vi "roboRIO v1.0 Reserve Relay.vi"(7 "Allow multiple opens?":bool, 8 "error in (no error)":errorcluster, 10 "Relay Channel List":T1) -> (0 "error out":errorcluster)   [LabVIEW 2021]
uses:
  <vilib>/myRIO/Common/Instrument Driver Framework/roboRIO v1.0/Relay/typedefs/Relay Channels List.ctl
  <vilib>/myRIO/Common/Instrument Driver Framework/roboRIO v1.0/Relay/typedefs/Relay Channels Enum.ctl
  <vilib>/myRIO/Common/Instrument Driver Framework/roboRIO v1.0/Resource Manager/vis/roboRIO v1.0 Reserve Channel.vi
  <vilib>/myRIO/Common/Instrument Driver Framework/roboRIO v1.0/Resource Manager/vis/roboRIO v1.0 Unreserve Channel.vi
  <vilib>/myRIO/Common/Instrument Driver Framework/roboRIO v1.0/Resource Manager/vis/roboRIO v1.0 Build Mutex Name.vi
  <vilib>/myRIO/Common/Instrument Driver Framework/Utilities/vis/IO Manager.vi
  <vilib>/Utility/error.llb/Error Cluster From Error Code.vi
  <vilib>/myRIO/Common/Instrument Driver Framework/Utilities/vis/Configuration Manager.vi
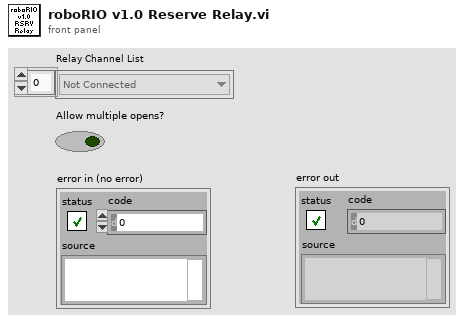
[diagram p1: front panel]
types:
  T1 = typedef "Relay Channels List.ctl" = T2[]
  T2 = typedef "Relay Channels Enum.ctl" = enum16{"Not Connected", "RELAY/RELAY0", "RELAY/RELAY1", "RELAY/RELAY2", "RELAY/RELAY3"}
  T3 = typedef "roboRIO v1.0 Channel Reservation List.ctl" = T4[]
  T4 = typedef "roboRIO v1.0 Channel Reservation Info.ctl" = cluster{"Channel Name":string, "Connector":T5, "Mutex ID":i32}
  T5 = typedef "roboRIO v1.0 Connector List.ctl" = enum32{"None", "ConnectorB", "ConnectorI2C", "ConnectorDIO", "ConnectorRSL", "ConnectorRELAY", "ConnectorAI", "ConnectorPWM", "ConnectorSPI"}
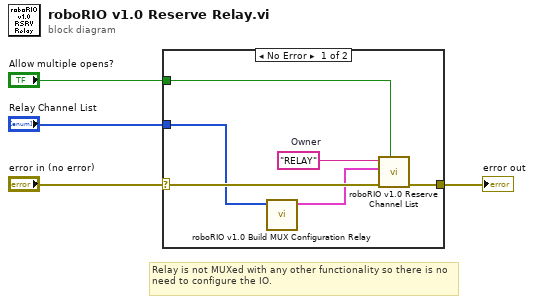
[diagram p0: block diagram]
diagram:
  # "Relay is not MUXed with any other functionality so there is no need to configure the IO."
  n1 = case shown="No Error" "error in (no error)" {
    selector: "error in (no error)" -> [w9 w11]
    tunnel: "Relay Channel List" -> [w6 _]
    tunnel: [w5 w11] -> w3
    tunnel: "Allow multiple opens?" -> [w10 _]
    frame No Error {
      w8 = "RELAY"  # Owner
      n2 = call <vilib>:"roboRIO v1.0 Build MUX Configuration Relay.vi"("Relay Channel List"=w6) -> ("Channel Reservation List"=w7:T3)  [unwired: 10 in]
      n3 = call <vilib>:"roboRIO v1.0 Reserve Channel List.vi"("Allow multiple opens?"=w10, "error in (no error)"=w9, "Channel Reservation List"=w7, "Owner"=w8) -> ("error out"=w5:errorcluster)  [unwired: 7 in]
    }
    frame Error {
    }
  }
  "error out" <- w3
